vi "IMAQdx HL-Snap.vi"(8 "ErrIn":errorcluster, 10 "ImgName":string="untitled", 11 "Camera":refnum<k21> caption="IMAQdx Session") -> (0 "ErrOut":errorcluster, 3 "ImgOut":T1)   [LabVIEW 2013]
doc: "Use this template to build a VI to use as a subVI."
uses:
  <vilib>/vision/Image Controls.llb/IMAQ Image.ctl
  <vilib>/vision/driver/NI_Vision_Acquisition_Software.lvlib
panel:
  # "Input Parameters"
  # "Output Parameters"
  # "VI Description:\nThis VI is created to snap a image from imaging device."
  # ":: MVI Framework V1.0 ::\nAuthor:Gaoke Yang\nEmail: gaoke.yang@yahoo.com\nWeb: www.mvicontrol.com\nCopyright (C) 2013, MVI Technologies All Rights Reserved"
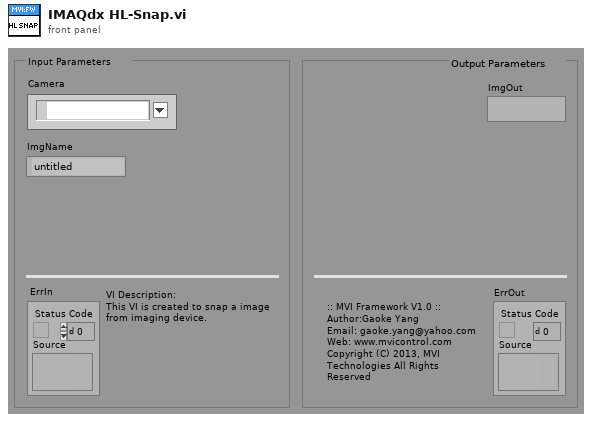
[diagram p1: front panel]
types:
  T1 = typedef "IMAQ Image.ctl" = refnum<image>
  T2 = typedef "IMAQdx.ctl" = refnum<k21>
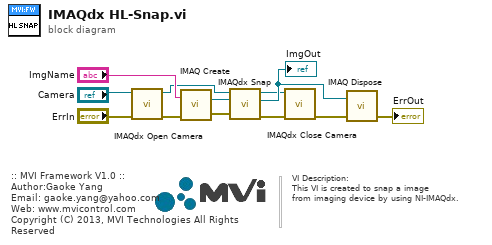
[diagram p0: block diagram]
diagram:
  # "VI Description:\nThis VI is created to snap a image\nfrom imaging device by using NI-IMAQdx."
  # ":: MVI Framework V1.0 ::\nAuthor:Gaoke Yang\nEmail: gaoke.yang@yahoo.com\nWeb: www.mvicontrol.com\nCopyright (C) 2013, MVI Technologies All Rights Reserved"
  n1 = call <vilib>:"IMAQdx Open Camera.vi"("error in"="ErrIn", "Session In"="Camera") -> ("error out"=w2:errorcluster, "Session Out"=w1:T2)  [unwired: 8 in]
  n2 = call "IMAQ Create"("Image Name"="ImgName", "error in (no error)"=w2) -> ("New Image"=w7:T1, "error out"=w6:errorcluster)  [unwired: 2 in, 1 out]
  n3 = call <vilib>:"IMAQdx Snap.vi"("error in"=w6, "Image In"=w7, "Session In"=w1) -> ("error out"=w3:errorcluster, "Image Out"=w8:T1, "Session Out"=w4:T2)  [unwired: 6 in]
  "ImgOut" <- w8
  n4 = call <vilib>:"IMAQdx Close Camera.vi"("error in"=w3, "Session In"=w4) -> ("error out"=w5:errorcluster)  [unwired: 9 in]
  n5 = call "IMAQ Dispose"("Image"=w8, "error in (no error)"=w5) -> ("error out"=→"ErrOut":errorcluster)  [unwired: 1 in, 3 out]
